vi "ErrorLog_ShowErrorDialog.vi"(5 "agent reference in":refnum<class "Agent.lvclass">, 7 "Owner (\"\"=All)":string, 8 "error in (no error)":errorcluster, 11 "reference in":refnum<class "ErrorLog.lvclass">) -> (0 "error out":errorcluster, 3 "reference out":refnum<class "ErrorLog.lvclass">)   [LabVIEW 2014, in "ErrorLog.lvclass"]
doc: "Shows Error Dialog"
uses:
  ErrorLog.lvclass
  <vilib>/addons/S5/ALOHA/Core/Agent/Agent.lvclass
panel:
  in  "pop":bool
  in  "CLR":bool
  out "Errors":string
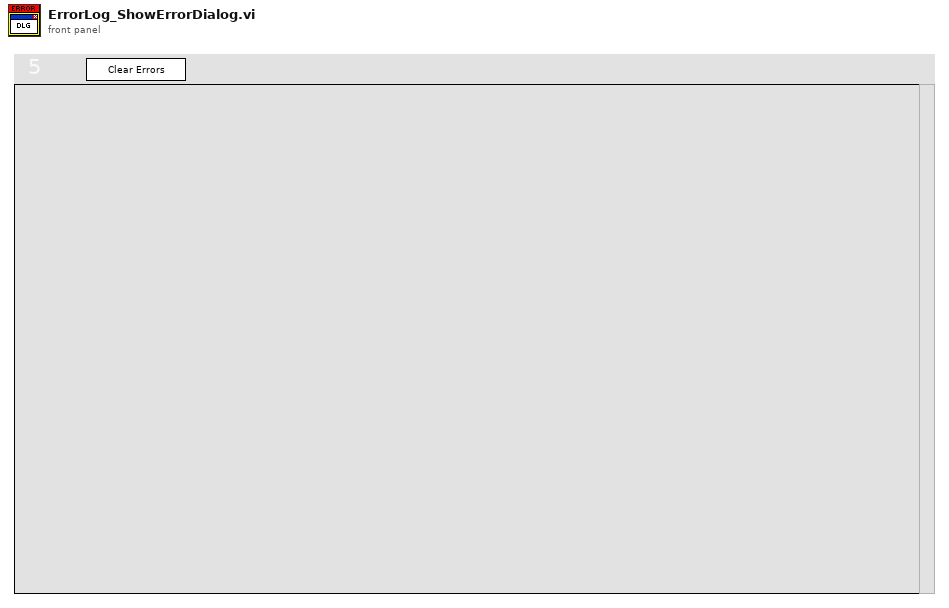
[diagram p1: front panel]
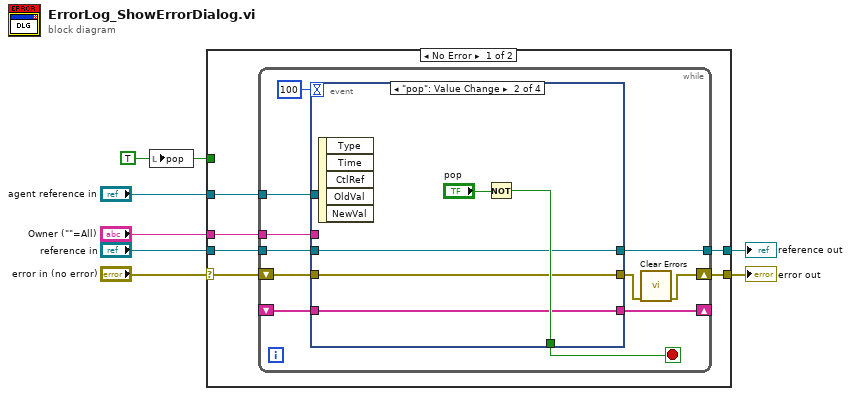
[diagram p0: block diagram]
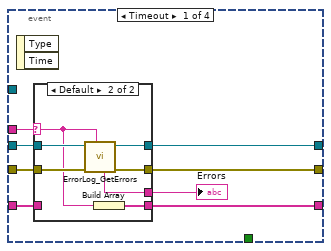
[diagram p2: hidden frame]
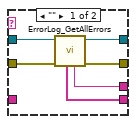
[diagram p3: hidden frame]
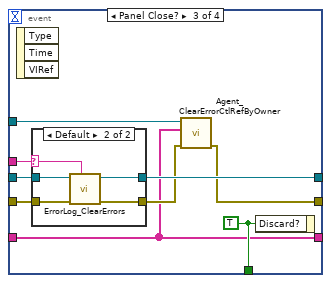
[diagram p4: hidden frame]
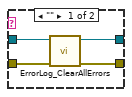
[diagram p5: hidden frame]
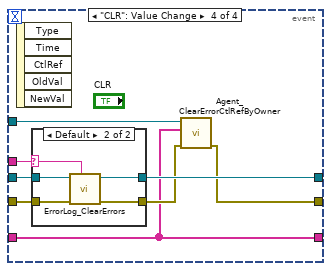
[diagram p6: hidden frame]
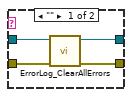
[diagram p7: hidden frame]
diagram:
  w5 = TRUE
  n1 = local write "pop"(w5) -> ()
  n2 = case shown="No Error" "error in (no error)" {
    selector: "error in (no error)" -> [w12 w86]
    tunnel: "reference in" -> [w13 w87]
    tunnel: w5 -> [_ _]
    tunnel: [w11 w87] -> w4
    tunnel: [w10 w86] -> w3
    tunnel: "Owner (\"\"=All)" -> [w9 _]
    tunnel: "agent reference in" -> [w8 _]
    frame No Error {
      n3 = while {
        shift-right: [w19] -> w10
        shift-left: w12 -> [w23]
        tunnel: w13 -> [w21]
        tunnel: [w20] -> w11
        tunnel: w9 -> [w17]
        shift-right: [w16] -> _
        shift-left: _ -> [w15]
        tunnel: w8 -> [w14]
        stop <- w22 stop-if-true
        n4 = event shown="[1] \"pop\": Value Change" {
          selector: _ -> [_ _ _ _]
          dyn-events: _ -> [_ _ _ _]
          timeout: 100 -> [_ _ _ _]
          tunnel: w23 -> [w32 w48 w57 w74]
          tunnel: [w30 w48 w53 w71] -> w18
          tunnel: [_ w49 w59 _] -> w22
          tunnel: w21 -> [w29 w47 w58 w75]
          tunnel: [w28 w47 w56 w73] -> w20
          tunnel: w17 -> [w27 _ w55 w76]
          tunnel: [w26 w46 w52 w70] -> w16
          tunnel: w15 -> [w25 w46 w52 w70]
          tunnel: w14 -> [_ _ w51 w69]
          event Timeout {
            n5 = event-data() -> ()  [unwired: 1 in, 2 out]
            n6 = case shown="Default" w27 {
              selector: w27 -> [_ w40]
              tunnel: w32 -> [w37 w45]
              tunnel: [w34 w44] -> w31
              tunnel: [w36 w43] -> w30
              tunnel: w29 -> [w38 w42]
              tunnel: [w35 w41] -> w28
              tunnel: [w33 w39] -> w26
              tunnel: w25 -> [_ _]
              frame "" {
                n7 = call-dynamic "ErrorLog_GetAllErrors.vi"("error in (no error)"=w37, "reference in"=w38) -> ("error out"=w36:errorcluster, "reference out"=w35:refnum<class "ErrorLog.lvclass">, "Errors since last clear"=w34:string, "Error owners since last clear"=w33:string[])  [unwired: 2 in, 4 out]
              }
              frame Default {
                n8 = call-dynamic "ErrorLog_GetErrors.vi"("Owner"=w40, "error in (no error)"=w45, "reference in"=w42) -> ("error out"=w43:errorcluster, "reference out"=w41:refnum<class "ErrorLog.lvclass">, "Errors since last clear"=w44:string)  [unwired: 3 in, 3 out]
                n9 = Build Array(w40) -> (w39:string[])
              }
            }
            "Errors" <- w31
          }
          event "pop": Value Change {
            n10 = event-data() -> ()  [unwired: 1 in, 5 out]
            n11 = Not(x="pop") -> (.not. x?=w49:bool)
          }
          event Panel Close? {
            w59 = TRUE ("Discard?")
            n12 = event-data() -> ()  [unwired: 1 in, 3 out]
            n13 = case shown="Default" w55 {
              selector: w55 -> [_ w64]
              tunnel: w58 -> [w63 w68]
              tunnel: w57 -> [w62 w67]
              tunnel: [w61 w66] -> w54
              tunnel: [w60 w65] -> w56
              frame "" {
                n14 = call-dynamic "ErrorLog_ClearAllErrors.vi"("error in (no error)"=w62, "reference in"=w63) -> ("error out"=w61:errorcluster, "reference out"=w60:refnum<class "ErrorLog.lvclass">)  [unwired: 8 in]
              }
              frame Default {
                n15 = call-dynamic "ErrorLog_ClearErrors.vi"("Owner"=w64, "error in (no error)"=w67, "reference in"=w68) -> ("error out"=w66:errorcluster, "reference out"=w65:refnum<class "ErrorLog.lvclass">)  [unwired: 7 in]
              }
            }
            n16 = call-dynamic "Agent_ClearErrorCtlRefByOwner.vi"("error in (no error)"=w54, "ErrorCtlRef Owners"=w52, "reference in"=w51) -> ("error out"=w53:errorcluster)  [unwired: 7 in, 1 out]
            n17 = event-data("Discard?"=w59) -> ()  [unwired: 1 in, 1 out]
          }
          event "CLR": Value Change {
            n18 = event-data() -> ()  [unwired: 1 in, 5 out]
            n19 = case shown="Default" w76 {
              selector: w76 -> [_ w81]
              tunnel: w75 -> [w80 w85]
              tunnel: w74 -> [w79 w84]
              tunnel: [w78 w83] -> w72
              tunnel: [w77 w82] -> w73
              frame "" {
                n20 = call-dynamic "ErrorLog_ClearAllErrors.vi"("error in (no error)"=w79, "reference in"=w80) -> ("error out"=w78:errorcluster, "reference out"=w77:refnum<class "ErrorLog.lvclass">)  [unwired: 8 in]
              }
              frame Default {
                n21 = call-dynamic "ErrorLog_ClearErrors.vi"("Owner"=w81, "error in (no error)"=w84, "reference in"=w85) -> ("error out"=w83:errorcluster, "reference out"=w82:refnum<class "ErrorLog.lvclass">)  [unwired: 7 in]
              }
            }
            n22 = call-dynamic "Agent_ClearErrorCtlRefByOwner.vi"("error in (no error)"=w72, "ErrorCtlRef Owners"=w70, "reference in"=w69) -> ("error out"=w71:errorcluster)  [unwired: 7 in, 1 out]
          }
        }
        n23 = call <vilib>:"Clear Errors.vi"("error in (no error)"=w18) -> ("error out"=w19:errorcluster)  [unwired: 5 in, 1 out]
      }
    }
    frame Error {
    }
  }
  "error out" <- w3
  "reference out" <- w4
